vi "Highlight String Constant.vi"(8 "error in (no error)":errorcluster, 10 "Cluster":T1, 11 "JKI SM in":refnum<class "JKI SM.lvclass">) -> (0 "error out":errorcluster, 3 "JKI SM out":refnum<class "JKI SM.lvclass">)   [LabVIEW 2020]
uses:
  JKI State Machine API/source/JKI SM/JKI SM.lvclass
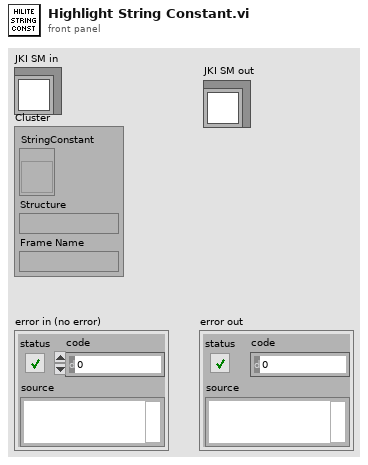
[diagram p1: front panel]
types:
  T1 = cluster{"StringConstant":refnum<vi>, "Structure":string, "Frame Name":string}
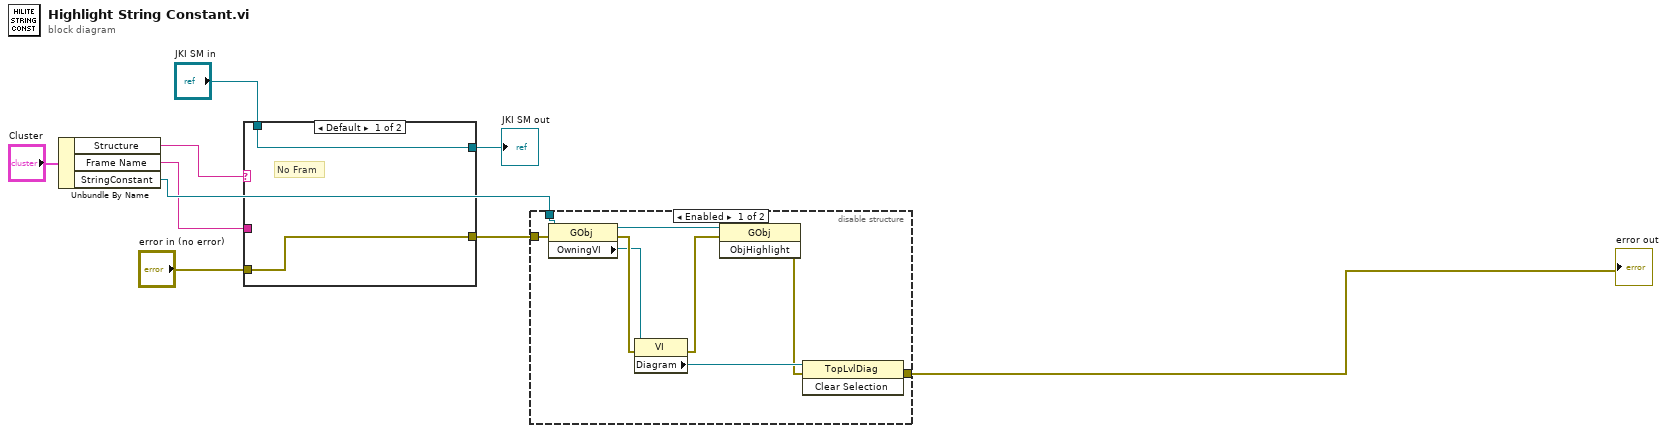
[diagram p0: block diagram]
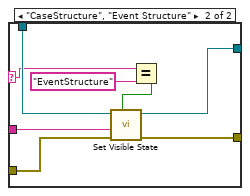
[diagram p2: hidden frame]
diagram:
  n1 = Unbundle By Name("Cluster") -> ("Structure"=w1:string, "Frame Name"=w2:string, "StringConstant"=w3:refnum<vi>)
  n2 = case shown="Default" w1 {
    selector: w1 -> [_ w13]
    tunnel: [w10 w19] -> w9
    tunnel: "error in (no error)" -> [w10 w18]
    tunnel: "JKI SM in" -> [w11 w17]
    tunnel: [w11 w16] -> w5
    tunnel: w2 -> [_ w15]
    frame Default {
      # "No Fram"
    }
    frame "CaseStructure", "Event Structure" {
      n3 = Equal?(x=w13, y="EventStructure") -> (x = y?=w12:bool)
      n4 = call "Set Visible State.vi"("Event Structure (F: Case Structure)"=w12, "error in (no error)"=w18, "State Name"=w15, "JKI SM in"=w17) -> ("error out"=w19:errorcluster, "JKI SM out"=w16:refnum<class "JKI SM.lvclass">)  [unwired: 6 in]
    }
  }
  "JKI SM out" <- w5
  n5 = disable-structure shown="Enabled" {
    disable-tunnel: w9 -> [w25 w29]
    disable-tunnel: [w23 w29] -> w4
    disable-tunnel: w3 -> [w20 _]
    frame Enabled {
      n6 = property class="GObj"(reference=w20, error in=w25) -> (reference out=w21:refnum<vi>, error out=w26:errorcluster, "OwningVI"=w24:refnum<vi>)
      n7 = property class="VI"(reference=w24, error in=w26) -> (error out=w27:errorcluster, "Diagram"=w28:refnum<vi>)  [unwired: 1 out]
      n8 = invoke class="GObj" method="ObjHighlight"(reference=w21, error in=w27) -> (error out=w22:errorcluster)  [unwired: 1 in, 2 out]
      n9 = invoke class="TopLvlDiag" method="Clear Selection"(reference=w28, error in=w22) -> (error out=w23:errorcluster)  [unwired: 1 in, 2 out]
    }
    frame Disabled {
    }
  }
  "error out" <- w4
